vi "REWORK_destroy_queues.vi"(8 "error_in":errorcluster, 11 "all_config_info":T1={"main_ini_file"={"SQL Driver"="", "SQL Server"="", "SQL Database"="", "SQL UID"="", "User table"="", "default language"="", "SCANNER COM port"=0, "SCANNER Baud rate"=0, "SCANNER Data bits"=0, "SCANNER Pairity"=enum."None", "SCANNER Stop bits"=10, "SCANNER Flow control"=0, "SCANNER Termination char"=0, "ST 140 name"="", "ST 140 listener IP"="", "ST 140 listener port"=0, "logout timeout [ms]"=0}, "SQL Password"="", "queue_refnums"={"MAIN_queue"=refnum, "SCANNER_queue"=refnum, "SCANNER_data"=refnum}} {"main_ini_file"."SCANNER Flow control" items=["None"=0, "XON/XOFF"=1, "RTS/CTS"=2, "DTR/DSR"=4]; "main_ini_file"."SCANNER Stop bits" items=["1.0"=10, "1.5"=15, "2.0"=20]}) -> (0 "error_out":errorcluster)   [LabVIEW 2019]
uses:
  ini/typedef/REWORK_all_config_info.ctl
  ini/typedef/REWORK_main_ini_file.ctl
  typedef/REWORK_queue_refnums.ctl
  typedef/REWORK_MAIN_queue_element.ctl
  MAIN/REWORK_MAIN_sequence_state.ctl
  typedef/REWORK_SCANNER_queue_element.ctl
  SCANNER/REWORK_SCANNER_sequence_state.ctl
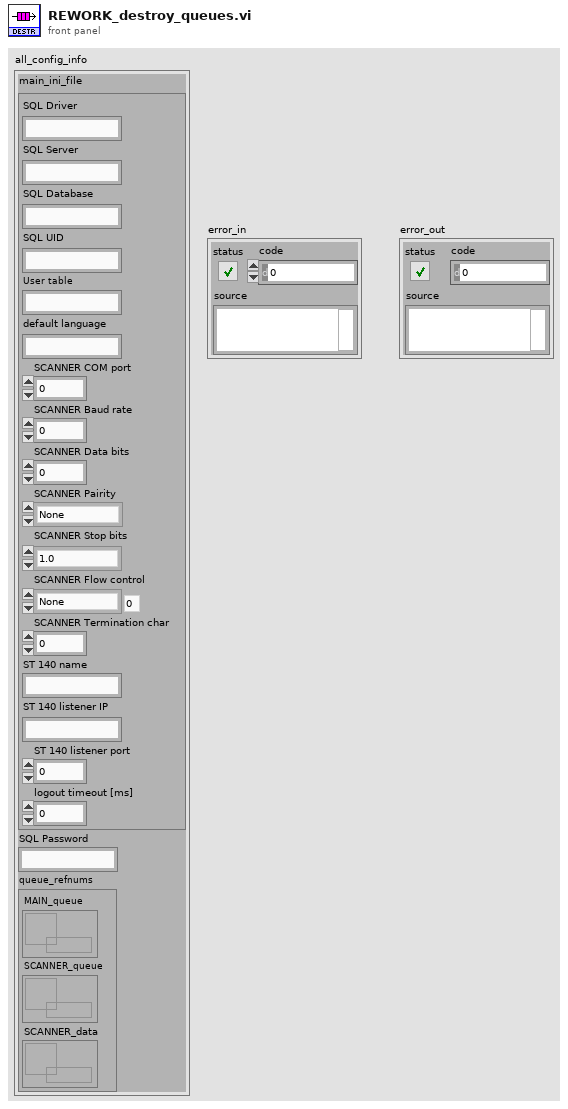
[diagram p1: front panel]
types:
  T1 = typedef "REWORK_all_config_info.ctl" = cluster{"main_ini_file":T2, "SQL Password":string, "queue_refnums":T3}
  T2 = typedef "REWORK_main_ini_file.ctl" = cluster{"SQL Driver":string, "SQL Server":string, "SQL Database":string, "SQL UID":string, "User table":string, "default language":string, "SCANNER COM port":u16, "SCANNER Baud rate":u32, "SCANNER Data bits":u16, "SCANNER Pairity":enum16{"None", "Odd", "Even", "Mark", "Space"}, "SCANNER Stop bits":u16, "SCANNER Flow control":u16, "SCANNER Termination char":u8, "ST 140 name":string, "ST 140 listener IP":string, "ST 140 listener port":u16, "logout timeout [ms]":i32}
  T3 = typedef "REWORK_queue_refnums.ctl" = cluster{"MAIN_queue":refnum<queue>, "SCANNER_queue":refnum<queue>, "SCANNER_data":refnum<queue>}
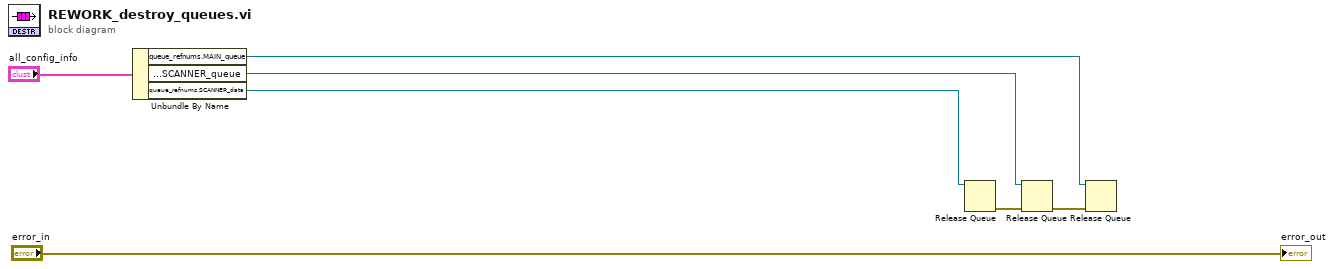
[diagram p0: block diagram]
diagram:
  n1 = Unbundle By Name("all_config_info") -> ("queue_refnums.MAIN_queue"=w1:refnum<queue>, "queue_refnums.SCANNER_queue"=w2:refnum<queue>, "queue_refnums.SCANNER_data"=w3:refnum<queue>)
  n2 = Release Queue(queue=w3) -> (error out=w5:errorcluster)  [unwired: 2 in, 2 out]
  n3 = Release Queue(queue=w2, error in (no error)=w5) -> (error out=w4:errorcluster)  [unwired: 1 in, 2 out]
  n4 = Release Queue(queue=w1, error in (no error)=w4) -> ()  [unwired: 1 in, 3 out]
  "error_out" <- "error_in"
